vi "ErasePreprocFile.vi"(8 "error in (no error)":errorcluster, 11 "Python in":refnum<class "Python.lvclass">) -> (0 "error out":errorcluster, 3 "Python out":refnum<class "Python.lvclass">)   [LabVIEW 2020, in "Python.lvclass"]
uses:
  Python.lvclass
  Python.lvclass/Python.ctl
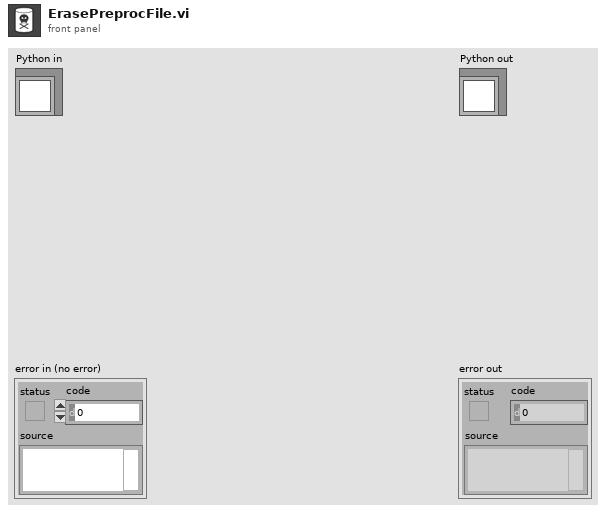
[diagram p1: front panel]
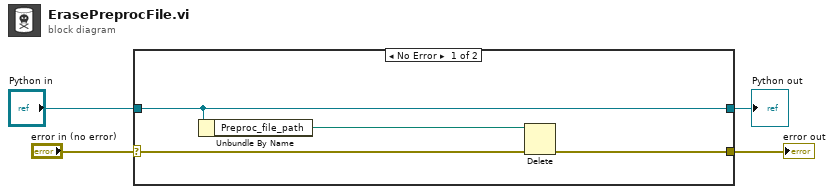
[diagram p0: block diagram]
diagram:
  n1 = case shown="No Error" "error in (no error)" {
    selector: "error in (no error)" -> [w6 w10]
    tunnel: [w5 w10] -> w3
    tunnel: [w8 w9] -> w1
    tunnel: "Python in" -> [w8 w9]
    frame No Error {
      n2 = Unbundle By Name(w8) -> ("Preproc_file_path"=w7:path)
      n3 = Delete(path (use dialog)=w7, error in=w6) -> (error out=w5:errorcluster)  [unwired: 3 in, 2 out]
    }
    frame Error {
    }
  }
  "error out" <- w3
  "Python out" <- w1
